vi "IP_Run.vi"(0 "Base Station":T5, 5 "Status":bool, 7 "Element":T4={"Cellular Tect"="", "IP_NETWORK"="BS1", "IP_TYPE"="", "IP_Client Address"="10.45.0.2", "IP_ThgroughPut(Mbps)"=0, "Duration"=0, "Status"=FALSE}, 11 "error in (no error)":errorcluster) -> (15 "error out":errorcluster)   [LabVIEW 2021]
uses:
  APIs/Controls/Base_Station_Emulator.ctl
  Controls/IP_Cellular Tech Type def.ctl
  Controls/IP_Network_Type def.ctl
  Controls/IP_Type-Tydedef.ctl
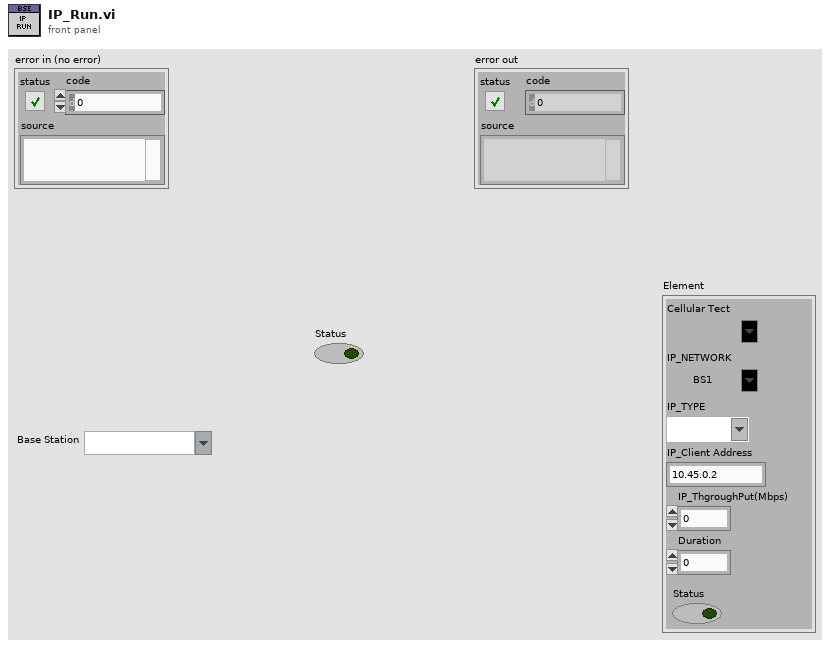
[diagram p1: front panel]
types:
  T1 = typedef "IP_Cellular Tech Type def.ctl" = string
  T2 = typedef "IP_Network_Type def.ctl" = string
  T3 = typedef "IP_Type-Tydedef.ctl" = string
  T4 = cluster{"Cellular Tect":T1, "IP_NETWORK":T2, "IP_TYPE":T3, "IP_Client Address":string, "IP_ThgroughPut(Mbps)":i32, "Duration":i32, "Status":bool}
  T5 = typedef "Base_Station_Emulator.ctl" = string
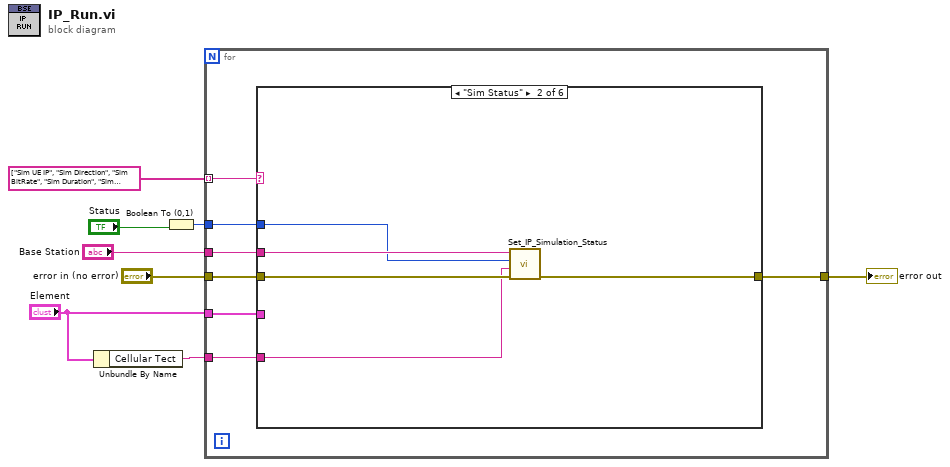
[diagram p0: block diagram]
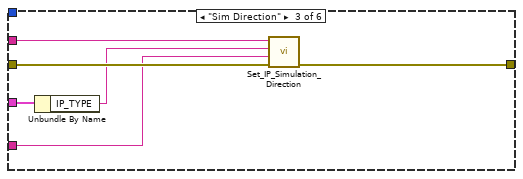
[diagram p3: hidden frame]
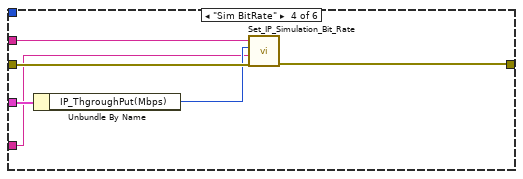
[diagram p4: hidden frame]
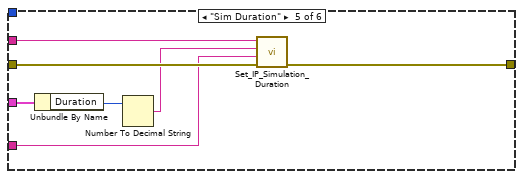
[diagram p5: hidden frame]
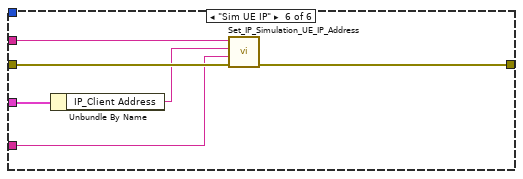
[diagram p6: hidden frame]
diagram:
  n1 = Unbundle By Name("Element") -> ("Cellular Tect"=w2:T1)
  n2 = Boolean To (0,1)(Boolean="Status") -> (0, 1=w3:i16)
  n3 = for {
    tunnel: "Element" -> [w15]
    tunnel: string[] ["Sim UE IP", "Sim Direction", "Sim BitRate", "Sim Duration", "Sim Status"] -> [w14] mode=indexing
    tunnel: w2 -> [w13]
    tunnel: "error in (no error)" -> [w12]
    tunnel: [w11] -> w6
    tunnel: "Base Station" -> [w10]
    tunnel: w3 -> [w9]
    n4 = case shown="\"Sim Status\"" w14 {
      tunnel: w15 -> [_ _ w24 w31 w36 w42]
      tunnel: w13 -> [_ w18 w23 w28 w37 w43]
      tunnel: w12 -> [w16 w21 w27 w33 w39 w46]
      tunnel: [w16 w20 w26 w32 w40 w45] -> w11
      tunnel: w10 -> [_ w19 w25 w29 w38 w44]
      tunnel: w9 -> [_ w17 _ _ _ _]
      frame Default {
      }
      frame "Sim Status" {
        n5 = call "Set_IP_Simulation_Status.vi"("error in (no error)"=w21, "Cellular Tech"=w18, "value"=w17, "Base Station"=w19) -> ("error out"=w20:errorcluster)  [unwired: 6 in, 1 out]
      }
      frame "Sim Direction" {
        n6 = Unbundle By Name(w24) -> ("IP_TYPE"=w22:T3)
        n7 = call "Set_IP_Simulation_Direction.vi"("error in (no error)"=w27, "Cellular Tech"=w23, "value"=w22, "Base Station"=w25) -> ("error out"=w26:errorcluster)  [unwired: 6 in, 1 out]
      }
      frame "Sim BitRate" {
        n8 = Unbundle By Name(w31) -> ("IP_ThgroughPut(Mbps)"=w30:i32)
        n9 = call "Set_IP_Simulation_Bit_Rate.vi"("error in (no error)"=w33, "Cellular Technology"=w28, "value"=w30, "Base Station"=w29) -> ("error out"=w32:errorcluster)  [unwired: 6 in, 1 out]
      }
      frame "Sim Duration" {
        n10 = Unbundle By Name(w36) -> ("Duration"=w35:i32)
        n11 = Number To Decimal String(number=w35) -> (decimal integer string=w34:string)  [unwired: 1 in]
        n12 = call "Set_IP_Simulation_Duration .vi"("error in (no error)"=w39, "Cellular Technology"=w37, "Value"=w34, "Base Station"=w38) -> ("error out"=w40:errorcluster)  [unwired: 6 in, 1 out]
      }
      frame "Sim UE IP" {
        n13 = Unbundle By Name(w42) -> ("IP_Client Address"=w41:string)
        n14 = call "Set_IP_Simulation_UE_IP_Address.vi"("error in (no error)"=w46, "Cellular Technology"=w43, "value"=w41, "Base Station"=w44) -> ("error out"=w45:errorcluster)  [unwired: 6 in, 1 out]
      }
    }
  }
  "error out" <- w6
